vi "ContMeasurement.vi"(8 "error in (no error)":errorcluster, 11 "TCP Network Connection in":refnum<k5>) -> (0 "error out":errorcluster, 3 "TCP Network Connection out":refnum<k5>)   [LabVIEW 2017]
panel:
  out "Sonstige Nachrichten":string[](array[string])
  out "Meas Result":dbl[](array[numeric])
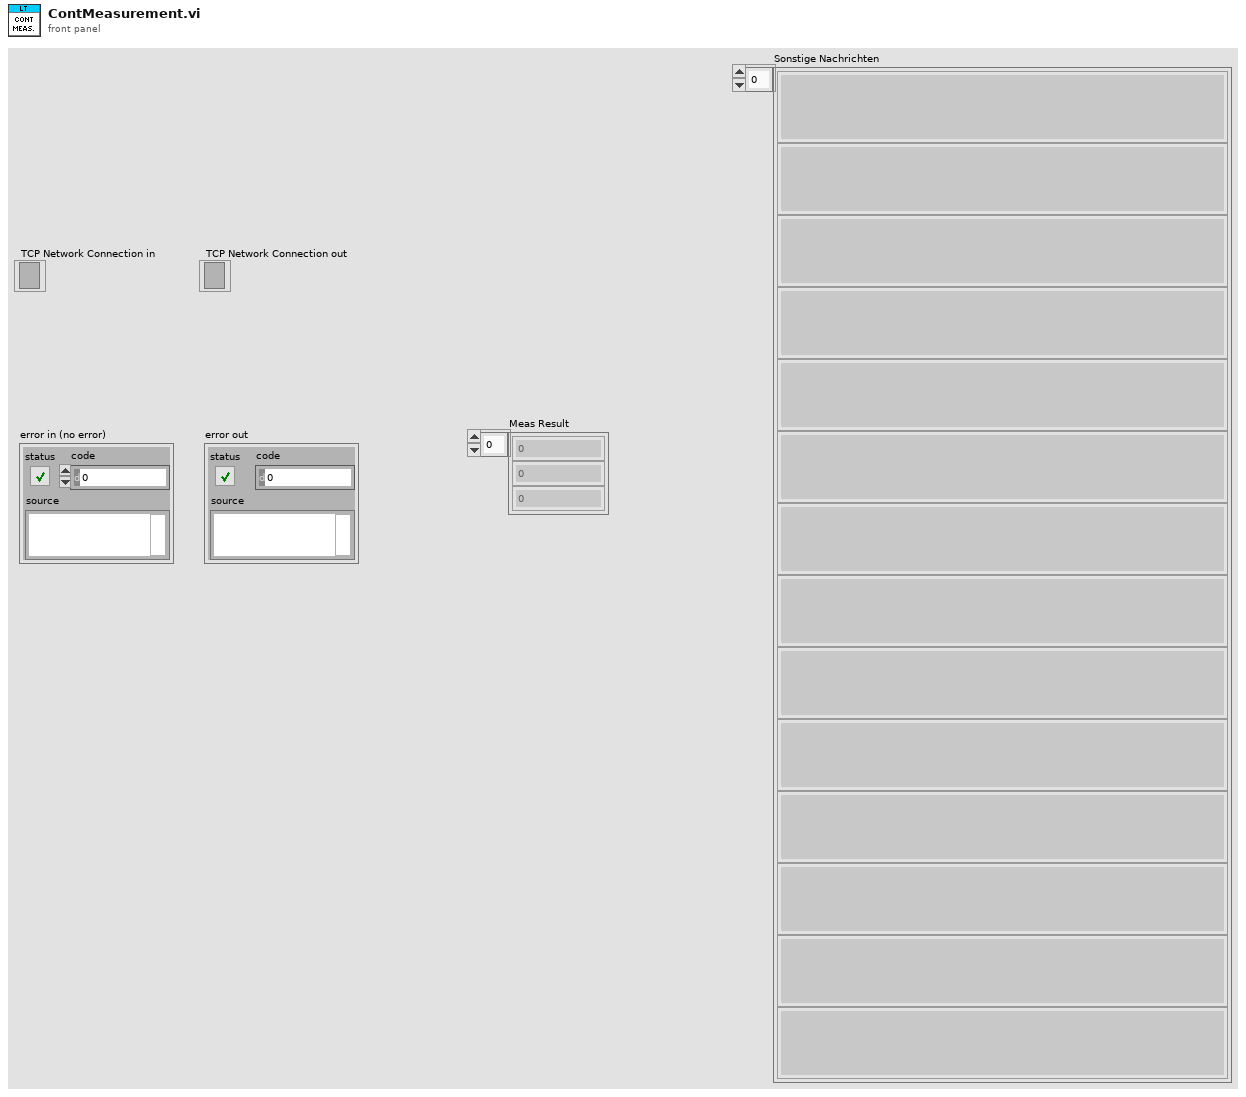
[diagram p1: front panel]
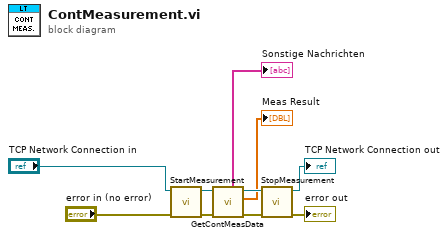
[diagram p0: block diagram]
diagram:
  n1 = call "StartMeasurement.vi"("error in (no error)"="error in (no error)", "TCP Network Connection in"="TCP Network Connection in") -> ("error out"=w7:errorcluster, "TCP Network Connection out"=w6:refnum<k5>)  [unwired: 6 in, 2 out]
  n2 = call "GetContMeasData.vi"("error in (no error)"=w7, "TCP Network Connection in"=w6) -> ("error out"=w3:errorcluster, "Meas Result"=→"Meas Result":dbl[], "TCP Network Connection out"=w5:refnum<k5>, "Sonstige Nachrichten"=→"Sonstige Nachrichten":string[])  [unwired: 6 in]
  n3 = call "StopMeasurement.vi"("error in (no error)"=w3, "TCP Network Connection in"=w5) -> ("error out"=→"error out":errorcluster, "TCP Network Connection out"=→"TCP Network Connection out":refnum<k5>)  [unwired: 6 in, 2 out]
